vi "ConsoleView Example.vi"() -> ()   [LabVIEW 2017, in "Logger Examples.lvlib"]
uses:
  Logger Examples.lvlib
  Source/ConsoleView/View/TypeDef/String Config.ctl
  Source/Composed Log/LoggerReference/LoggerReference.lvclass/LoggerReference.ctl
  Source/ConsoleView/ConsoleInterface/ConsoleSession.lvclass/ConsoleSession.ctl
  Source/Composed Log/Types/Log Level.ctl
  428adf5f-c5ee-4c09-9a5b-736284a89f6a.vi
  428adf5f-c5ee-4c09-9a5b-736284a89f6a.vi/739c411a-770b-41f8-82cd-699df0492461.vi
  Source/Composed Log/LoggerReference/Return Aggregate Queues.vi
  Source/Composed Log/LoggerReference/Add Aggregate Log.vi
  428adf5f-c5ee-4c09-9a5b-736284a89f6a.vi/739c411a-770b-41f8-82cd-699df0492461.vi/83f1a723-0147-4a0d-b8f7-8c03f11df13a.vi
  Source/Composed Log/LoggerReference/Log.vi
  Source/Composed Log/LoggerReference/Get Valid Event Time.vi
  Source/Composed Log/LoggerReference/Send Add Sink.vi
  Source/Composed Log/LoggerReference/Remove Stale Logs.vi
  Source/ConsoleView/Sink/ConsoleSink.lvclass
  C:/CS/Internal/LabVIEW/Logger/Source/Composed Log/Log Sink/Log Sink.lvclass
  Source/Composed Log/Application Logger/Launch Worker Loop.vi
  Source/Composed Log/LoggerReference/Initialize Logger Instance.vi
  Source/Composed Log/Singleton Event Log/Logger Queue FGV.vi
  Source/Composed Log/IErrorFormat/IErrorFormat.lvclass
  Source/Composed Log/LoggerReference/LoggerReference.lvclass
  Source/Composed Log/Log Sink/Log Sink.lvclass
  Source/Composed Log/Singleton Event Log/Singleton Event Log.lvlib
  Source/Composed Log/Composed Log.lvlib
  Source/ConsoleView/ConsoleInterface/ConsoleSession.lvclass
  Source/ConsoleView/View/ConsoleView.lvclass
panel:
  in  "Timeout Event Rate (ms)":u32=250 min=1
  in  "Hide":bool
  in  "Show":bool
  in  "Event Level":T1(ring)
  in  "Data To Log":string
  in  "Source":string="User"
  in  "Log":bool
  # "Run the VI. \n\nUse the controls to log custom messages."
  # "Show or hide the viewer. See block diagram for details."
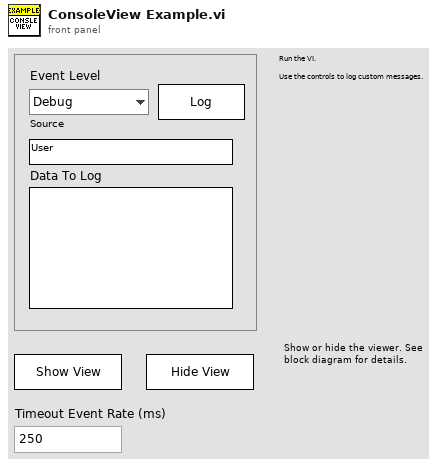
[diagram p1: front panel]
types:
  T1 = enum16{"Debug", "Info", "Warning", "Error", "Critical"}
  T2 = typedef "ConsoleView.lvlib/ConsoleView.lvclass/String Config.ctl" = cluster{"BG Color":u32, "Text Color":u32, "Font Size":u32, "Bold?":bool}
  T3 = typedef "Composed Log.lvlib/Log Level.ctl" = enum16{"Debug", "Info", "Warning", "Error", "Critical"}
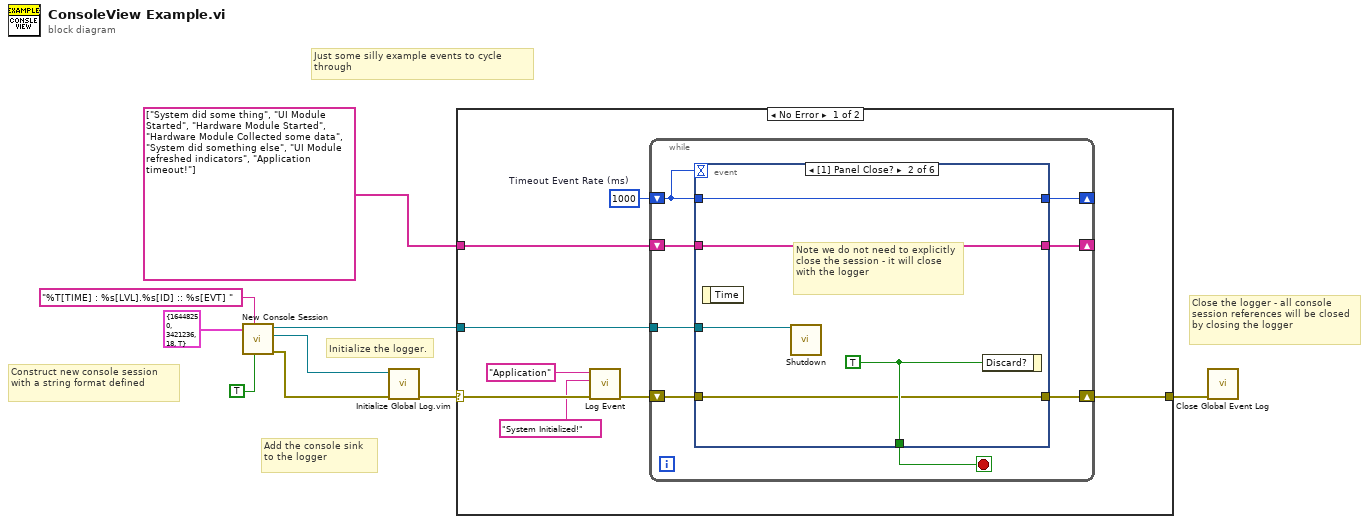
[diagram p0: block diagram]
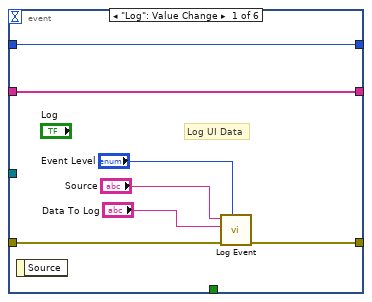
[diagram p2: hidden frame]
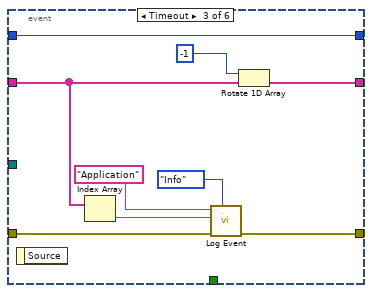
[diagram p3: hidden frame]
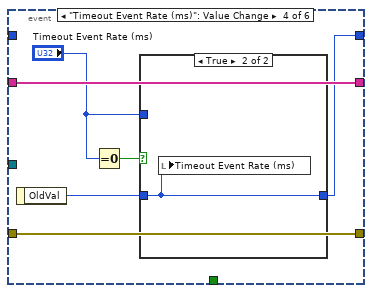
[diagram p4: hidden frame]
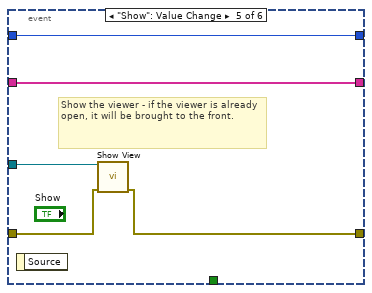
[diagram p6: hidden frame]
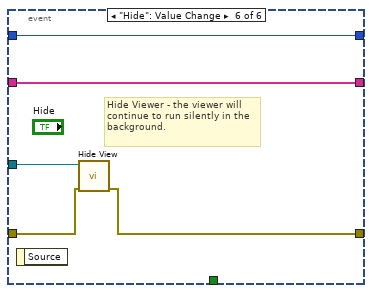
[diagram p7: hidden frame]
diagram:
  # "Construct new console session with a string format defined"
  # "Just some silly example events to cycle through"
  # "Add the console sink to the logger"
  # "Close the logger - all console session references will be closed by closing the logger"
  # "Initialize the logger."
  n1 = call "New Console Session.vi"("Persist After Shutdown?(F)"=TRUE, "Format Specifier"="%T[TIME] : %s[LVL].%s[ID] :: %s[EVT] ", "UI Config"=T2 {"BG Color"=16448250, "Text Color"=3421236, "Font Size"=18, "Bold?"=TRUE}) -> ("error out"=w4:errorcluster, "ConsoleSink out"=w7:refnum<class "ConsoleSink.lvclass">, "ConsoleSession out"=w6:refnum<class "ConsoleSession.lvclass">)  [unwired: 6 in]
  n2 = call "Initialize Global Log.vim"("error in (no error)"=w4, "Log Sink(s)"=w7) -> ("error out"=w9:errorcluster)  [unwired: 8 in, 1 out]
  n3 = case shown="No Error" w9 {
    selector: w9 -> [w15 w65]
    tunnel: [w10 w65] -> w8
    tunnel: w6 -> [w17 _]
    tunnel: string[] ["System did some thing", "UI Module Started", "Hardware Module Started", "Hardware Module Collected some data", "System did something else", "UI Module refreshed indicators", "Application timeout!"] -> [w12 _]
    frame No Error {
      w16 = 1000  # Timeout Event Rate (ms)
      n4 = call "Log Event.vi"("error in (no error)"=w15, "Data To Log"="System Initialized!", "SourceID"="Application") -> ("error out"=w11:errorcluster)  [unwired: 8 in]
      n5 = while {
        tunnel: w17 -> [w24]
        shift-right: [w23] -> _
        shift-left: w16 -> [w22]
        shift-right: [w20] -> _
        shift-left: w12 -> [w21]
        shift-right: [w18] -> w10
        shift-left: w11 -> [w19]
        stop <- w25 stop-if-true
        n6 = event shown="[1] Panel Close?" {
          selector: _ -> [_ _ _ _ _ _]
          dyn-events: _ -> [_ _ _ _ _ _]
          timeout: w22 -> [_ _ _ _ _ _]
          tunnel: [_ w37 _ _ _ _] -> w25
          tunnel: w24 -> [_ w33 _ _ w59 w64]
          tunnel: [w29 w36 w45 w48 w58 w63] -> w23
          tunnel: w22 -> [w29 w36 w45 _ w58 w63]
          tunnel: w21 -> [w28 w35 w43 w52 w57 w62]
          tunnel: [w28 w35 w42 w52 w57 w62] -> w20
          tunnel: w19 -> [w27 w34 w39 w51 w56 w61]
          tunnel: [w26 w34 w38 w51 w55 w60] -> w18
          event "Log": Value Change {
            # "Log UI Data"
            n7 = event-data() -> ()  [unwired: 1 in, 1 out]
            n8 = call "Log Event.vi"("Event Level"="Event Level", "error in (no error)"=w27, "Data To Log"="Data To Log", "SourceID"="Source") -> ("error out"=w26:errorcluster)  [unwired: 7 in]
          }
          event Panel Close? {
            w37 = TRUE ("Discard?")
            # "Note we do not need to explicitly close the session - it will close with the logger"
            n9 = event-data() -> ()  [unwired: 1 in, 1 out]
            n10 = call "Shutdown.vi"("ConsoleInterface in"=w33) -> ()  [unwired: 10 in, 1 out]
            n11 = event-data("Discard?"=w37) -> ()  [unwired: 1 in, 1 out]
          }
          event Timeout {
            n12 = event-data() -> ()  [unwired: 1 in, 1 out]
            n13 = Index Array(array=w43) -> (element=w44:string)  [unwired: 1 in]
            n14 = call "Log Event.vi"("Event Level"=Log_Level."Info", "error in (no error)"=w39, "Data To Log"=w44, "SourceID"="Application") -> ("error out"=w38:errorcluster)  [unwired: 7 in]
            n15 = Rotate 1D Array(1:w43, 2:-1 ("n")) -> (0:w42:string[])
          }
          event "Timeout Event Rate (ms)": Value Change {
            n16 = event-data() -> ("OldVal"=w49:u32)  [unwired: 1 in]
            n17 = Equal To 0?(x="Timeout Event Rate (ms)") -> (x = 0?=w50:bool)
            n18 = case shown="True" w50 {
              tunnel: w49 -> [_ w54]
              tunnel: [w53 w54] -> w48
              tunnel: "Timeout Event Rate (ms)" -> [w53 _]
              frame False {
              }
              frame True {
                n19 = local write "Timeout Event Rate (ms)"(w54) -> ()
              }
            }
          }
          event "Show": Value Change {
            # "Show the viewer - if the viewer is already open, it will be brought to the front."
            n20 = event-data() -> ()  [unwired: 1 in, 1 out]
            n21 = call "Show View.vi"("error in (no error)"=w56, "ConsoleInterface in"=w59) -> ("error out"=w55:errorcluster)  [unwired: 8 in, 1 out]
          }
          event "Hide": Value Change {
            # "Hide Viewer - the viewer will continue to run silently in the background."
            n22 = event-data() -> ()  [unwired: 1 in, 1 out]
            n23 = call "Hide View.vi"("error in (no error)"=w61, "ConsoleInterface in"=w64) -> ("error out"=w60:errorcluster)  [unwired: 8 in, 1 out]
          }
        }
      }
    }
    frame Error {
      # "This shouldn't occur, but if it does just stop instead of leaving the example user confused about why the VI is running but log events aren't working."
    }
  }
  n24 = call "Close Global Event Log.vi"("error in (no error)"=w8) -> ()  [unwired: 10 in, 1 out]
